vi "BonOMM-SAOMM.Test.vi"() -> ()   [LabVIEW 2011] (continued)
                n3227 = Array To Spreadsheet String(delimiter (Tab)="\n", array=w7372, 3:"%5f") -> (spreadsheet string=w7370:string)
                n3228 = Get Date/Time String(date format (0)=enum16{"short", "long", "abbreviated"}."short", want seconds? (F)=TRUE) -> (date string=w7356:string, time string=w7351:string)  [unwired: 1 in]
                n3229 = local read "path_syslogs"() -> (w7366:path)
                n3230 = Search and Replace String(replace all?=TRUE ("replace all? (F)"), input string=w7356, search string="-") -> (result string=w7350:string)  [unwired: 5 in, 3 out]
                n3231 = Search and Replace String(replace all?=TRUE ("replace all? (F)"), input string=w7351, search string=":") -> (result string=w7349:string)  [unwired: 5 in, 3 out]
                n3232 = Concatenate Strings(w7368, "\n\n***\n\n", w7370) -> (w7367:string)
                n3233 = Concatenate Strings(w7350, w7349, ".lvdt" ("name or relative path")) -> (w7359:string)
                n3234 = Build Path(base path=w7366, name or relative path="LVDTs") -> (appended path=w7364:path)
                n3235 = local read "File I/O Error"() -> (w7358:errorcluster)
                n3236 = Build Path(base path=w7364, name or relative path=w7359) -> (appended path=w7363:path)
                n3237 = Write to Text File(file (use dialog)=w7363, text=w7367, error in=w7358) -> (error out=w7357:errorcluster)  [unwired: 1 in, 2 out]
                n3238 = local write "File I/O Error"(w7357) -> ()
              }
              event "SpliterSelector": Value Change {
                n3239 = event-data() -> ("OldVal"=w7375:u16, "NewVal"=w7374:u16)  [unwired: 1 in, 3 out]
                n3240 = Not Equal?(x=w7375, y=w7374) -> (x != y?=w7373:bool)
                n3241 = case shown="True" w7373 {
                  frame False {
                  }
                  frame True {
                    n3242 = flat-sequence {
                      frame #0 {
                        "SplitterMoving" <- TRUE
                      }
                      frame #1 {
                        n3243 = flat-sequence {
                          tunnel: "SpliterSelector" -> [w7382]
                          frame #0 {
                            n3244 = case shown="1" w7382 {
                              tunnel: [w7383 w7388 w7389] -> _
                              frame 2 {
                                w7385 = u16 1 items=["Initialisation", "Mise dans le faisceau", "Retirer du faisceau"] ("Commande")
                                n3245 = local read "Splitter VRN"() -> (w7384:refnum<visa-resource-name>)
                                n3246 = call "MicroSlide-Execute.vi"("VISA resource name"=w7384, "Commande"=w7385) -> ("Error OUT"=w7383:errorcluster)  [unwired: 10 in, 3 out]
                              }
                              frame 0, Default {
                                w7386 = u16 0 items=["Initialisation", "Mise dans le faisceau", "Retirer du faisceau"] ("Commande")
                                n3247 = local read "Splitter VRN"() -> (w7387:refnum<visa-resource-name>)
                                n3248 = call "MicroSlide-Execute.vi"("VISA resource name"=w7387, "Commande"=w7386) -> ("Error OUT"=w7388:errorcluster)  [unwired: 10 in, 3 out]
                              }
                              frame 1 {
                                w7391 = u16 2 items=["Initialisation", "Mise dans le faisceau", "Retirer du faisceau"] ("Commande")
                                n3249 = local read "Splitter VRN"() -> (w7390:refnum<visa-resource-name>)
                                n3250 = call "MicroSlide-Execute.vi"("VISA resource name"=w7390, "Commande"=w7391) -> ("Error OUT"=w7389:errorcluster)  [unwired: 10 in, 3 out]
                              }
                            }
                          }
                          frame #1 {
                            n3251 = local write "SplitterMoving"(FALSE ("SplitterMoving")) -> ()
                          }
                        }
                        n3252 = while {
                          stop <- w7381 continue-if-true
                          n3253 = local read "SpliterIndic"() -> (w7378:bool)
                          n3254 = Wait (ms)(milliseconds to wait=u32 250) -> ()  [unwired: 1 out]
                          n3255 = Not(x=w7378) -> (.not. x?=→"SpliterIndic":bool)
                          n3256 = local read "SplitterMoving"() -> (w7381:bool)
                        }
                      }
                      frame #2 {
                        # "À mettre en gestion d'erreur"
                        n3257 = local write "SpliterIndic"(TRUE ("SpliterIndic")) -> ()
                      }
                    }
                  }
                }
              }
            }
          }
          "Événements Usagés" <- w956
          n3258 = while {
            stop <- w991 stop-if-true
            # "Boucle d'analyse d'image à haute fréquence ..."
            n3259 = event shown="[1] \"ProcessImage\": Value Change" {
              selector: _ -> [_ _]
              dyn-events: _ -> [_ _]
              timeout: 50 -> [_ _]
              event Timeout {
                n3260 = event-data() -> ()  [unwired: 1 in, 2 out]
              }
              event "ProcessImage": Value Change {
                n3261 = event-data() -> ()  [unwired: 1 in, 5 out]
                n3262 = local read "ROIXOffset"() -> (w999:u16)
                n3263 = local read "ROIYOffset"() -> (w995:u16)
                n3264 = local write "ProcessImage"(FALSE) -> ()
                n3265 = local read "XCentroid"() -> (w1000:dbl)
                n3266 = local read "YCentroid"() -> (w996:dbl)
                n3267 = local read "ImageBuffer"() -> (w1012:u16[][])
                n3268 = local read "MaskObjet"() -> (w1013:u8[][])
                n3269 = To Double Precision Float(number=w999) -> (double precision float=w998:dbl)
                n3270 = To Double Precision Float(number=w995) -> (double precision float=w997:dbl)
                n3271 = Subtract(x=w1000, y=w998) -> (x-y=w993:dbl)
                n3272 = Subtract(x=w996, y=w997) -> (x-y=w994:dbl)
                n3273 = local read "PixScale1"() -> (w1015:dbl)
                n3274 = local read "Binning"() -> (w1016:u16)
                n3275 = call "SAOMM-ROI-Stats.vi"("ImageBuffer"=w1012, "ObjectMask"=w1013, "intervals"=32) -> ("ROI Histogram"=→"Histogramme de la ROI":T10, "ImageStat"=w1009:T2)  [unwired: 11 in]
                "ImageStat" <- w1009
                n3276 = To Long Integer(number=w1012) -> (32bit integer=w1002:i32[][])
                n3277 = To Double Precision Float(number=w1016) -> (double precision float=w1014:dbl)
                n3278 = Multiply(x=w1015, y=w1014) -> (x*y=w1004:dbl)
                n3279 = call "PSF-Fitting.vi"("Centoid X"=w993, "Centroid Y"=w994, "ROI"=w1002, "''/pix"=w1004) -> ("Credible?"=w992:bool, "PSF Graph"=w1001:cluster{"PSF X":dbl[], "PSF Y":dbl[]}[], "Seeing"=w1003:dbl)  [unwired: 8 in, 1 out]
                n3280 = case shown="False" w992 {
                  tunnel: w1001 -> [_ w1025]
                  tunnel: w1003 -> [_ w1024]
                  tunnel: [w1019 w1025] -> w1011
                  tunnel: [inf w1024] -> w1010
                  frame False {
                    n3281 = Build Array(0.0) -> (w1021:dbl[])
                    n3282 = Bundle(w1021, w1021) -> (w1020:cluster{dbl[], dbl[]})  [unwired: 1 in]
                    n3283 = Build Array(w1020, w1020) -> (w1019:cluster{dbl[], dbl[]}[])
                  }
                  frame True {
                  }
                }
                "PSF Graph" <- w1011
                "Seeing" <- w1010
                n3284 = Unbundle By Name(w1009) -> ("ObjectMaximumValue"=w1008:dbl)
                n3285 = Greater?(x=w1008, y=50000.0) -> (0:w1006:bool)
                n3286 = property on="Saturé" class="Bool (strict)"("Blinking"=w1006, "Visible"=w1006) -> ()  [unwired: 2 in, 2 out]
              }
            }
            n3287 = local read "Quit"() -> (w991:bool)
          }
          n3288 = control-ref of="PrAMS actif"() -> (w958:refnum<vi>)
          n3289 = Tick Count (ms)() -> (millisecond timer value=w959:u32)
          n3290 = Tick Count (ms)() -> (millisecond timer value=w960:u32)
          n3291 = control-ref of="HexaCons actif"() -> (w957:refnum<vi>)
          n3292 = while {
            tunnel: [w1369] -> w949
            i -> [w1370]
            stop <- w1369 stop-if-true
            n3293 = event shown="[0] Timeout" {
              selector: _ -> [_ _ _ _ _ _ _ _ _ _ _ _ _ _ _ _ _ _ _ _ _ _ _]
              dyn-events: _ -> [_ _ _ _ _ _ _ _ _ _ _ _ _ _ _ _ _ _ _ _ _ _ _]
              timeout: 200 -> [_ _ _ _ _ _ _ _ _ _ _ _ _ _ _ _ _ _ _ _ _ _ _]
              tunnel: w1370 -> [w1378 _ _ _ _ _ _ _ _ _ _ _ _ _ _ _ _ _ _ _ _ _ _]
              event Timeout {
                # "À passer dans une boucle à part ?"
                n3294 = event-data() -> ()  [unwired: 1 in, 2 out]
                n3295 = local read "Integrating"() -> (w1375:bool)
                n3296 = Quotient & Remainder(x=w1378, y=25) -> (x-y*floor(x/y)=w1376:i32)  [unwired: 1 out]
                n3297 = Equal To 0?(x=w1378) -> (x = 0?=w1380:bool)
                n3298 = Equal To 0?(x=w1376) -> (x = 0?=w1374:bool)
                n3299 = Not(x=w1375) -> (.not. x?=w1373:bool)
                n3300 = And(x=w1374, y=w1373) -> (x .and. y?=w1372:bool)
                n3301 = Or(x="FalconRefresh", y=w1380) -> (x .or. y?=w1385:bool)
                n3302 = Equal?(x=w1378, y=1) -> (x = y?=w1382:bool)
                n3303 = Compound Arithmetic op=OR(w1382, "HexapodRefresh", w1372) -> (w1379:bool)
                n3304 = case shown="False" w1385 {
                  frame False {
                  }
                  frame True {
                    n3305 = Tick Count (ms)() -> (millisecond timer value=→"FalconQuery":u32)
                    n3306 = local write "FalconRefresh"(FALSE ("Refresh")) -> ()
                    n3307 = local read "PrAMS VRN"() -> (w1402:refnum<visa-resource-name>)
                    n3308 = local read "PrAMS Error"() -> (w1404:errorcluster)
                    n3309 = local read "MessageType"() -> (w1399:cluster{string[], u32[]})
                    n3310 = control-ref of="PrAMS actif"() -> (w1400:refnum<vi>)
                    n3311 = local read "Signature"() -> (w1398:u32)
                    n3312 = call "SAOMM-QueryFalcon.vi"("PRAMMS-COMM IN"=w1402, "Bool Refnum"=w1400, "Signature"=w1398, "Error IN"=w1404, "CommandCluster"=w1399) -> ("PRAMMS-COMM OUT"=w1401:refnum<visa-resource-name>, "Error OUT"=w1403:errorcluster)  [unwired: 9 in]
                    n3313 = local write "PrAMS Error"(w1403) -> ()
                    n3314 = local write "PrAMS VRN"(w1401) -> ()
                    "QueryingPraMS" <- TRUE
                  }
                }
                n3315 = case shown="False" w1379 {
                  frame False {
                  }
                  frame True {
                    n3316 = local write "HexapodRefresh"(FALSE ("Refresh")) -> ()
                    n3317 = Tick Count (ms)() -> (millisecond timer value=→"HexapodQuery":u32)
                    n3318 = local read "MessageType"() -> (w1391:cluster{string[], u32[]})
                    n3319 = control-ref of="HexaCons actif"() -> (w1387:refnum<vi>)
                    n3320 = local read "PrAMS Error"() -> (w1393:errorcluster)
                    n3321 = local read "Signature"() -> (w1390:u32)
                    n3322 = call "SAOMM-QueryHexapod.vi"("PRAMMS-COMM IN"="Hexapod VRN", "Bool Refnum"=w1387, "Signature"=w1390, "Error IN"=w1393, "EnumMessageType"=w1391) -> ("PRAMMS-COMM OUT"=w1388:refnum<visa-resource-name>, "Error OUT"=w1392:errorcluster)  [unwired: 9 in]
                    n3323 = local write "PrAMS Error"(w1392) -> ()
                    n3324 = local write "Hexapod VRN"(w1388) -> ()
                    "QueryingHexapod" <- TRUE ("Refresh")
                  }
                }
              }
              event "refresh": Value Change {
                n3325 = event-data() -> ()  [unwired: 1 in, 5 out]
                n3326 = case shown="True" "refresh" {
                  frame False {
                  }
                  frame True {
                    n3327 = flat-sequence {
                      frame #0 {
                        n3328 = local read "MessageType"() -> (w1414:cluster{string[], u32[]})
                        n3329 = control-ref of="PrAMS actif"() -> (w1413:refnum<vi>)
                        n3330 = local read "PrAMS VRN"() -> (w1412:refnum<visa-resource-name>)
                        n3331 = local read "PrAMS Error"() -> (w1411:errorcluster)
                        n3332 = local read "Signature"() -> (w1410:u32)
                        n3333 = call "SAOMM-SendGET.vi"("PRAMMS-COMM IN"=w1412, "Bool Refnum"=w1413, "MessageType"=w1414, "Signature"=w1410, "Error IN"=w1411, "Active GET"="GetCommand") -> ("PRAMMS-COMM OUT"=w1409:refnum<visa-resource-name>, "Error OUT"=w1408:errorcluster)  [unwired: 8 in]
                        n3334 = local write "PrAMS Error"(w1408) -> ()
                        n3335 = local write "PrAMS VRN"(w1409) -> ()
                      }
                      frame #1 {
                        n3336 = local write "refresh"(FALSE) -> ()
                      }
                    }
                  }
                }
              }
              event "Mode": Value Change {
                # "C'est ici qu'on changera les mutex pour les boutons quand ceux-ci seront définis ..."
                n3337 = event-data() -> ("OldVal"=w1417:u16, "NewVal"=w1416:u16)  [unwired: 1 in, 3 out]
                n3338 = case shown="2" w1417 {
                  frame 0, Default {
                    # "On passe de 'Opération fixe' à ..."
                  }
                  frame 1 {
                    # "On passe de 'Asservissement passif' à ..."
                  }
                  frame 2 {
                    # "On passe de 'Asservissement actif' à ..."
                  }
                  frame 3 {
                    # "On passe de 'Calibration' à ..."
                  }
                }
                n3339 = case shown="3" w1416 {
                  frame 0, Default {
                    # "... 'Opération fixe'"
                  }
                  frame 1 {
                    # "'Asservissement passif'"
                  }
                  frame 2 {
                    # "'Asservissement actif'"
                  }
                  frame 3 {
                    # "'Calibration'"
                  }
                }
              }
              event "ImgArray": Mouse Down {
                n3340 = event-data() -> ("Coords"=w1422:T48)  [unwired: 1 in, 6 out]
                n3341 = local read "Integrating"() -> (w1420:bool)
                n3342 = local read "Servo"() -> (w1419:bool)
                n3343 = Not(x=w1419) -> (.not. x?=w1418:bool)
                n3344 = And(x=w1420, y=w1418) -> (x .and. y?=w1421:bool)
                n3345 = case shown="True" w1421 {
                  tunnel: w1422 -> [_ w1457]
                  tunnel: w1418 -> [w1423 _]
                  frame False {
                    n3346 = case shown="False" w1423 {
                      frame False {
                        n3347 = One Button Dialog(message="Vous ne pouvez pas modifier la ROI pendant l'asservissement") -> ()  [unwired: 1 in, 1 out]
                      }
                      frame True {
                      }
                    }
                  }
                  frame True {
                    n3348 = control-ref of="ImgArray"() -> (w1454:refnum<vi>)
                    n3349 = local read "ROIWidth"() -> (w1453:u16)
                    n3350 = local read "ROIHeight"() -> (w1452:u16)
                    n3351 = call "Click2CursorPosition.vi"("reference"=w1454, "ClickPosition"=w1457) -> ("CursorX"=w1456:dbl, "CursorY"=w1455:dbl)  [unwired: 12 in]
                    n3352 = call "SAOMM-Cursor2ROI.vi"("ImgRef"=w1454, "CursorX"=w1456, "CursorY"=w1455, "ROIWidth"=w1453, "ROIHeight"=w1452) -> ("XÉtoile"=w1430:dbl, "YÉtoile"=w1429:dbl, "ROIXOffset"=w1434:u16, "ROIYOffset"=w1433:u16)  [unwired: 7 in]
                    n3353 = local write "YROIRef"(w1430) -> ()
                    n3354 = local write "XROIRef"(w1429) -> ()
                    n3355 = local write "ROIXOffset"(w1434) -> ()
                    n3356 = local write "ROIYOffset"(w1433) -> ()
                    n3357 = local read "Binning"() -> (w1443:u16)
                    n3358 = local read "ROIWidth"() -> (w1436:u16)
                    n3359 = local read "ROIHeight"() -> (w1437:u16)
                    n3360 = local read "Naxis1"() -> (w1441:u16)
                    n3361 = local read "Naxis2"() -> (w1440:u16)
                    n3362 = Bundle("XÉtoile"=w1430, "YÉtoile"=w1429) -> (w1435:cluster{"XÉtoile":dbl, "YÉtoile":dbl})  [unwired: 1 in]
                    n3363 = Bundle("Naxis1"=w1441, "Naxis2"=w1440) -> (w1442:cluster{"Naxis1":u16, "Naxis2":u16})  [unwired: 1 in]
                    n3364 = Bundle("ROIWidth"=w1436, "ROIHeight"=w1437) -> (w1439:cluster{"ROIWidth":u16, "ROIHeight":u16})  [unwired: 1 in]
                    n3365 = Bundle("ROIXOffset"=w1434, "ROIYOffset"=w1433) -> (w1438:cluster{"ROIXOffset":u16, "ROIYOffset":u16})  [unwired: 1 in]
                    n3366 = local read "MessageType"() -> (w1445:cluster{string[], u32[]})
                    n3367 = control-ref of="PrAMS-ACK"() -> (w1446:refnum<vi>)
                    n3368 = control-ref of="PrAMS actif"() -> (w1451:refnum<vi>)
                    n3369 = local read "PrAMS VRN"() -> (w1450:refnum<visa-resource-name>)
                    n3370 = local read "PrAMS Error"() -> (w1449:errorcluster)
                    n3371 = call "SAOMM-ROI_Fixer.vi"("Binning"=w1443, "Use Offset?"=TRUE, "naxis"=w1442, "ROI"=w1439, "Offset"=w1438, "Reference Pixel"=w1435) -> ("FixedOffset"=w1427:cluster{"ROIXOffset":u16, "ROIYOffset":u16}, "FixedPixel"=w1428:cluster{"PixelX":dbl, "PixelY":dbl})  [unwired: 6 in, 2 out]
                    n3372 = Unbundle By Name(w1428) -> ("PixelX"=w1426:dbl, "PixelY"=w1425:dbl)
                    n3373 = call "SAOMM-UpdateROI.vi"("PRAMMS-COMM IN"=w1450, "Active Refnum"=w1451, "PrAMS-ACK"=w1446, "MessageType"=w1445, "Error IN"=w1449, "Position"=w1427) -> ("PRAMMS-COMM OUT"=w1448:refnum<visa-resource-name>, "Error OUT"=w1447:errorcluster)  [unwired: 7 in, 1 out]
                    n3374 = local write "PrAMS Error"(w1447) -> ()
                    n3375 = local write "PrAMS VRN"(w1448) -> ()
                    n3376 = property on="ImgArray" class="IntGraph (strict)"() -> ("Cursor.Cursor Position"=w1432:T44)  [unwired: 2 in, 2 out]
                    n3377 = local write "XReference"(w1426) -> ()
                    n3378 = local write "YReference"(w1425) -> ()
                    n3379 = Bundle(cluster=w1432, "Cursor X"=w1426, "Cursor Y"=w1425) -> (w1431:T44)
                    n3380 = property on="ImgArray" class="IntGraph (strict)"("Cursor.Cursor Position"=w1431) -> ()  [unwired: 2 in, 2 out]
                  }
                }
              }
              event "ClearDump": Value Change {
                # "Tout ceci est du débuggage ..."
                n3381 = event-data() -> ()  [unwired: 1 in, 5 out]
                n3382 = local write "nDumped"(0 ("nDumped")) -> ()
                n3383 = local write "Dump"("") -> ()
              }
              event "ImageFPS": Value Change {
                n3384 = event-data() -> ()  [unwired: 1 in, 5 out]
                n3385 = flat-sequence {
                  tunnel: [w1462] -> w1461
                  tunnel: [w1465] -> w1460
                  tunnel: w1461 -> [w1465]
                  tunnel: w1460 -> [w1477]
                  frame #0 {
                    n3386 = Tick Count (ms)() -> (millisecond timer value=w1462:u32)
                  }
                  frame #1 {
                    n3387 = local read "MessageType"() -> (w1468:cluster{string[], u32[]})
                    n3388 = control-ref of="PrAMS actif"() -> (w1470:refnum<vi>)
                    n3389 = control-ref of="PrAMS-ACK"() -> (w1469:refnum<vi>)
                    n3390 = local read "PrAMS Error"() -> (w1471:errorcluster)
                    n3391 = local read "PrAMS VRN"() -> (w1472:refnum<visa-resource-name>)
                    n3392 = local read "ImageFPS"() -> (w1463:dbl)
                    n3393 = local read "Signature"() -> (w1464:u32)
                    n3394 = call-poly "SAOMM-Num2littleEndian.vi"("Number"=w1463) -> ("LiitleEndianedData"=w1466:u8[])  [unwired: 14 in]
                    n3395 = call "SAOMM-SendSET.vi"("PRAMMS-COMM IN"=w1472, "Active Refnum"=w1470, "PrAMS-ACK"=w1469, "Signature"=w1464, "Error IN"=w1471, "MessageType"=w1468, "Active SET"="emtSetImageDisplayFrameRate", "Value (little endianed byte array)"=w1466) -> ("PRAMMS-COMM OUT"=w1474:refnum<visa-resource-name>, "Error OUT"=w1473:errorcluster)  [unwired: 4 in, 2 out]
                    n3396 = local write "PrAMS Error"(w1473) -> ()
                    n3397 = local write "PrAMS VRN"(w1474) -> ()
                  }
                  frame #2 {
                    n3398 = Tick Count (ms)() -> (millisecond timer value=w1476:u32)
                    n3399 = Subtract(x=w1476, y=w1477) -> (x-y=→"SetFPSTime":u32)
                  }
                }
              }
              event "exptime": Value Change {
                n3400 = event-data() -> ()  [unwired: 1 in, 5 out]
                n3401 = flat-sequence {
                  tunnel: [w1480] -> w1479
                  tunnel: [w1482] -> w1478
                  tunnel: w1479 -> [w1482]
                  tunnel: w1478 -> [w1497]
                  frame #0 {
                    n3402 = Tick Count (ms)() -> (millisecond timer value=w1480:u32)
                  }
                  frame #1 {
                    n3403 = local read "MessageType"() -> (w1488:cluster{string[], u32[]})
                    n3404 = control-ref of="PrAMS actif"() -> (w1490:refnum<vi>)
                    n3405 = control-ref of="PrAMS-ACK"() -> (w1489:refnum<vi>)
                    n3406 = local read "PrAMS Error"() -> (w1491:errorcluster)
                    n3407 = local read "PrAMS VRN"() -> (w1492:refnum<visa-resource-name>)
                    n3408 = expression code="x*1000"("exptime") -> (w1484:dbl)
                    n3409 = local read "Signature"() -> (w1481:u32)
                    n3410 = To Unsigned Long Integer(number=w1484) -> (unsigned 32bit integer=w1483:u32)
                    n3411 = call-poly "SAOMM-Num2littleEndian.vi"("Number"=w1483) -> ("LiitleEndianedData"=w1486:u8[])  [unwired: 14 in]
                    n3412 = call "SAOMM-SendSET.vi"("PRAMMS-COMM IN"=w1492, "Active Refnum"=w1490, "PrAMS-ACK"=w1489, "Signature"=w1481, "Error IN"=w1491, "MessageType"=w1488, "Active SET"="emtSetImageExposureTime", "Value (little endianed byte array)"=w1486) -> ("PRAMMS-COMM OUT"=w1494:refnum<visa-resource-name>, "Error OUT"=w1493:errorcluster)  [unwired: 4 in, 2 out]
                    n3413 = local write "PrAMS Error"(w1493) -> ()
                    n3414 = local write "PrAMS VRN"(w1494) -> ()
                  }
                  frame #2 {
                    n3415 = Tick Count (ms)() -> (millisecond timer value=w1496:u32)
                    n3416 = Subtract(x=w1496, y=w1497) -> (x-y=→"SetExpTime":u32)
                  }
                }
              }
              event "FPGA Value": Value Change {
                n3417 = event-data() -> ("NewVal"=w1501:u16)  [unwired: 1 in, 4 out]
                n3418 = local read "Integrating"() -> (w1498:bool)
                n3419 = local read "Servo"() -> (w1499:bool)
                n3420 = Or(x=w1499, y=w1498) -> (x .or. y?=w1500:bool)
                n3421 = case shown="False" w1500 {
                  tunnel: w1501 -> [w1506 _]
                  frame False {
                    n3422 = Number To Decimal String(number=w1506) -> (decimal integer string=w1505:string)  [unwired: 1 in]
                    n3423 = call-poly "SAOMM-Num2littleEndian.vi"("Number"=w1506) -> ("LiitleEndianedData"=w1509:u8[])  [unwired: 14 in]
                    n3424 = local read "MessageType"() -> (w1512:cluster{string[], u32[]})
                    n3425 = control-ref of="PrAMS actif"() -> (w1514:refnum<vi>)
                    n3426 = control-ref of="PrAMS-ACK"() -> (w1513:refnum<vi>)
                    n3427 = local read "PrAMS VRN"() -> (w1516:refnum<visa-resource-name>)
                    n3428 = local read "PrAMS Error"() -> (w1515:errorcluster)
                    n3429 = control-ref of="TERMINAL"() -> (w1507:refnum<vi>)
                    n3430 = control-ref of="Indicateur d'état"() -> (w1508:refnum<vi>)
                    n3431 = local read "Signature"() -> (w1510:u32)
                    n3432 = Concatenate Strings("FAPG.set -> (", w1505, ")") -> (w1503:string)
                    n3433 = call "TERMINAL.vi"("Indicateur Refnum"=w1508, "Terminal Refnum"=w1507, "Indicateur d'état"=w1503) -> ()
                    n3434 = call "SAOMM-SendSET.vi"("PRAMMS-COMM IN"=w1516, "Active Refnum"=w1514, "PrAMS-ACK"=w1513, "Signature"=w1510, "Error IN"=w1515, "MessageType"=w1512, "Active SET"="emtSetFPGACtrl", "Value (little endianed byte array)"=w1509) -> ("PRAMMS-COMM OUT"=w1518:refnum<visa-resource-name>, "Error OUT"=w1517:errorcluster)  [unwired: 4 in, 2 out]
                    n3435 = local write "PrAMS Error"(w1517) -> ()
                    n3436 = local write "PrAMS VRN"(w1518) -> ()
                  }
                  frame True {
                    n3437 = One Button Dialog(message="Impossible de modifier le FPGActrl pendant que la caméra fonctionne") -> ()  [unwired: 1 in, 1 out]
                  }
                }
              }
              event "Binning": Value Change {
                n3438 = event-data() -> ("OldVal"=w1524:u16, "NewVal"=w1523:u16)  [unwired: 1 in, 3 out]
                n3439 = local read "Integrating"() -> (w1521:bool)
                n3440 = local read "Servo"() -> (w1520:bool)
                n3441 = Or(x=w1521, y=w1520) -> (x .or. y?=w1522:bool)
                n3442 = case shown="False" w1522 {
                  tunnel: w1524 -> [w1536 _]
                  tunnel: w1523 -> [w1534 _]
                  frame False {
                    w1548 = "cam_Binning "
                    # "Passer dans une astrométrie ?"
                    n3443 = flat-sequence {
                      tunnel: [w1581] -> w1564
                      tunnel: [w1597] -> w1563
                      tunnel: w1564 -> [w1597]
                      tunnel: w1535 -> [w1589]
                      tunnel: w1533 -> [w1588]
                      tunnel: w1532 -> [w1587]
                      tunnel: [w1586] -> w1562
                      tunnel: [w1585] -> w1561
                      tunnel: [w1584] -> w1560
                      tunnel: w1563 -> [w1611]
                      tunnel: [w1608] -> w1531
                      tunnel: w1562 -> [w1608]
                      tunnel: w1561 -> [w1607]
                      tunnel: w1560 -> [w1602]
                      frame #0 {
                        n3444 = Tick Count (ms)() -> (millisecond timer value=w1581:u32)
                      }
                      frame #1 {
                        n3445 = local read "MessageType"() -> (w1591:cluster{string[], u32[]})
                        n3446 = control-ref of="PrAMS-ACK"() -> (w1582:refnum<vi>)
                        n3447 = control-ref of="PrAMS actif"() -> (w1583:refnum<vi>)
                        n3448 = local read "Signature"() -> (w1590:u32)
                        n3449 = local read "PrAMS VRN"() -> (w1596:refnum<visa-resource-name>)
                        n3450 = local read "PrAMS Error"() -> (w1595:errorcluster)
                        n3451 = call "SAOMM-BinningFixer.vi"("PRAMMS-COMM IN"=w1596, "Active Refnum"=w1583, "PrAMS-ACK"=w1582, "Signature"=w1590, "SendSET"=TRUE, "MessageType"=w1591, "Error IN"=w1595, "Binning"=w1589, "NAXIS"=w1587, "ROI Sizes"=w1588) -> ("PRAMMS-COMM OUT"=w1594:refnum<visa-resource-name>, "ScaleFactor"=w1586:dbl, "ROISizesOut"=w1585:T49, "ROIMinMax"=w1584:T50, "Error OUT"=w1593:errorcluster)  [unwired: 1 in]
                        n3452 = local write "PrAMS Error"(w1593) -> ()
                        n3453 = local write "PrAMS VRN"(w1594) -> ()
                      }
                      frame #2 {
                        n3454 = Tick Count (ms)() -> (millisecond timer value=w1610:u32)
                        n3455 = Subtract(x=w1610, y=w1611) -> (x-y=→"SetBinningTime":u32)
                        n3456 = Unbundle(w1607) -> ("ROIXOffset OUT"=w1606:u16, "ROIYOffset OUT"=w1605:u16, "ROIWidth OUT"=w1604:u16, "ROIHeight OUT"=w1603:u16)
                        n3457 = Unbundle(w1602) -> ("ROIXMin"=→"ROIXMin":u16, "ROIYXMax"=→"ROIXMax":u16, "ROIYMin"=→"ROIYMin":u16, "ROIYMax"=→"ROIYMax":u16)
                        n3458 = local write "ROIXOffset"(w1606) -> ()
                        n3459 = local write "ROIYOffset"(w1605) -> ()
                        n3460 = local write "ROIWidth"(w1604) -> ()
                        n3461 = local write "ROIHeight"(w1603) -> ()
                      }
                    }
                    n3462 = local read "Naxis1"() -> (w1525:u16)
                    n3463 = local read "Naxis2"() -> (w1526:u16)
                    n3464 = local read "ROIXOffset"() -> (w1530:u16)
                    n3465 = local read "ROIYOffset"() -> (w1529:u16)
                    n3466 = local read "ROIWidth"() -> (w1528:u16)
                    n3467 = local read "ROIHeight"() -> (w1527:u16)
                    n3468 = Bundle("OldVal"=w1536, "NewVal"=w1534) -> (w1535:cluster{"OldVal":u16, "NewVal":u16})  [unwired: 1 in]
                    n3469 = Bundle("Naxis1"=w1525, "Naxis2"=w1526) -> (w1532:cluster{"Naxis1":u16, "Naxis2":u16})  [unwired: 1 in]
                    n3470 = Bundle("ROIXOffset"=w1530, "ROIYOffset"=w1529, "ROIWidth"=w1528, "ROIHeight"=w1527) -> (w1533:T51)  [unwired: 1 in]
                    n3471 = property on="ImgArray" class="IntGraph (strict)"() -> ("Cursor.Cursor X"=w1559:dbl, "Cursor.Cursor Y"=w1558:dbl)  [unwired: 2 in, 2 out]
                    n3472 = case shown="2" w1534 {
                      tunnel: [TRUE FALSE FALSE FALSE] -> w1540
                      tunnel: [FALSE TRUE FALSE FALSE] -> w1539
                      tunnel: [FALSE FALSE TRUE FALSE] -> w1538
                      tunnel: [FALSE FALSE FALSE TRUE] -> w1537
                      frame 1, Default {
                      }
                      frame 2 {
                      }
                      frame 4 {
                      }
                      frame 5 {
                      }
                    }
                    n3473 = Multiply(x=w1531, y=w1559) -> (x*y=w1557:dbl)
                    n3474 = Multiply(x=w1558, y=w1531) -> (x*y=w1556:dbl)
                    n3475 = Round To Nearest(number=w1557) -> (nearest integer value=w1555:dbl)
                    n3476 = Round To Nearest(number=w1556) -> (nearest integer value=w1554:dbl)
                    n3477 = Current VI's Menubar() -> (w1553:refnum<k9>)
                    n3478 = Concatenate Strings(w1548, "1x1" ("string")) -> (w1549:string)
                    n3479 = Set Menu Item Info(6:w1540, 7:w1549, 11:w1553) -> (3:w1552:refnum<k9>)  [unwired: 4 in, 1 out]
                    n3480 = Concatenate Strings(w1548, "2x2" ("string")) -> (w1543:string)
                    n3481 = Set Menu Item Info(6:w1539, 7:w1543, 11:w1552) -> (3:w1551:refnum<k9>)  [unwired: 4 in, 1 out]
                    n3482 = local write "YReference"(w1554) -> ()
                    n3483 = local write "XReference"(w1555) -> ()
                    n3484 = Concatenate Strings(w1548, "4x4" ("string")) -> (w1542:string)
                    n3485 = Set Menu Item Info(6:w1538, 7:w1542, 11:w1551) -> (3:w1550:refnum<k9>)  [unwired: 4 in, 1 out]
                    n3486 = Concatenate Strings(w1548, "5x5" ("string")) -> (w1541:string)
                    n3487 = property on="ImgArray" class="IntGraph (strict)"("Cursor.Cursor X"=w1555, "Cursor.Cursor Y"=w1554) -> ()  [unwired: 2 in, 2 out]
                    n3488 = Set Menu Item Info(6:w1537, 7:w1541, 11:w1550) -> ()  [unwired: 4 in, 2 out]
                  }
                  frame True {
                  }
                }
              }
              event "EMGain": Value Change {
                n3489 = event-data() -> ("NewVal"=w1615:u16)  [unwired: 1 in, 4 out]
                n3490 = local read "Integrating"() -> (w1613:bool)
                n3491 = local read "Servo"() -> (w1614:bool)
                n3492 = Or(x=w1614, y=w1613) -> (x .or. y?=w1612:bool)
                n3493 = case shown="False" w1612 {
                  tunnel: w1615 -> [w1616 _]
                  frame False {
                    n3494 = call-poly "SAOMM-Num2littleEndian.vi"("Number"=w1616) -> ("LiitleEndianedData"=w1617:u8[])  [unwired: 14 in]
                    n3495 = local read "MessageType"() -> (w1620:cluster{string[], u32[]})
                    n3496 = control-ref of="PrAMS actif"() -> (w1622:refnum<vi>)
                    n3497 = control-ref of="PrAMS-ACK"() -> (w1621:refnum<vi>)
                    n3498 = local read "PrAMS VRN"() -> (w1624:refnum<visa-resource-name>)
                    n3499 = local read "PrAMS Error"() -> (w1623:errorcluster)
                    n3500 = local read "Signature"() -> (w1618:u32)
                    n3501 = call "SAOMM-SendSET.vi"("PRAMMS-COMM IN"=w1624, "Active Refnum"=w1622, "PrAMS-ACK"=w1621, "Signature"=w1618, "Error IN"=w1623, "MessageType"=w1620, "Active SET"="emtSetImageEMGain", "Value (little endianed byte array)"=w1617) -> ("PRAMMS-COMM OUT"=w1626:refnum<visa-resource-name>, "Error OUT"=w1625:errorcluster)  [unwired: 4 in, 2 out]
                    n3502 = local write "PrAMS Error"(w1625) -> ()
                    n3503 = local write "PrAMS VRN"(w1626) -> ()
                  }
                  frame True {
                  }
                }
              }
              event "GoCam": Value Change {
                n3504 = event-data() -> ()  [unwired: 1 in, 5 out]
                n3505 = flat-sequence {
                  tunnel: [w1630] -> w1628
                  tunnel: [w1633] -> w1627
                  tunnel: w1628 -> [w1633]
                  tunnel: w1627 -> [w1644]
                  frame #0 {
                    n3506 = local write "GoCam"(FALSE ("GoCam")) -> ()
                    n3507 = Tick Count (ms)() -> (millisecond timer value=w1630:u32)
                  }
                  frame #1 {
                    # "emtStartAcquisition ne prend pas d'arguments"
                    n3508 = local read "MessageType"() -> (w1635:cluster{string[], u32[]})
                    n3509 = control-ref of="PrAMS actif"() -> (w1637:refnum<vi>)
                    n3510 = control-ref of="PrAMS-ACK"() -> (w1636:refnum<vi>)
                    n3511 = local read "PrAMS Error"() -> (w1638:errorcluster)
                    n3512 = local read "PrAMS VRN"() -> (w1639:refnum<visa-resource-name>)
                    n3513 = local read "Signature"() -> (w1631:u32)
                    n3514 = call "SAOMM-SendSET.vi"("PRAMMS-COMM IN"=w1639, "Active Refnum"=w1637, "PrAMS-ACK"=w1636, "Signature"=w1631, "Error IN"=w1638, "MessageType"=w1635, "Active SET"="emtStartAcquisition", "Value (little endianed byte array)"=u8[] []) -> ("PRAMMS-COMM OUT"=w1641:refnum<visa-resource-name>, "Error OUT"=w1640:errorcluster)  [unwired: 4 in, 2 out]
                    n3515 = local write "PrAMS Error"(w1640) -> ()
                    n3516 = local write "PrAMS VRN"(w1641) -> ()
                  }
                  frame #2 {
                    n3517 = Tick Count (ms)() -> (millisecond timer value=w1643:u32)
                    n3518 = Subtract(x=w1643, y=w1644) -> (x-y=→"StartTime":u32)
                  }
                }
              }
              event "StopCam": Value Change {
                n3519 = event-data() -> ()  [unwired: 1 in, 5 out]
                n3520 = flat-sequence {
                  tunnel: [w1648] -> w1646
                  tunnel: [w1651] -> w1645
                  tunnel: w1646 -> [w1651]
                  tunnel: w1645 -> [w1662]
                  frame #0 {
                    n3521 = local write "StopCam"(FALSE ("StopCam")) -> ()
                    n3522 = Tick Count (ms)() -> (millisecond timer value=w1648:u32)
                  }
                  frame #1 {
                    # "emtStartAcquisition ne prend pas d'arguments"
                    n3523 = local read "PrAMS VRN"() -> (w1657:refnum<visa-resource-name>)
                    n3524 = control-ref of="PrAMS-ACK"() -> (w1654:refnum<vi>)
                    n3525 = local read "PrAMS Error"() -> (w1656:errorcluster)
                    n3526 = local read "MessageType"() -> (w1653:cluster{string[], u32[]})
                    n3527 = control-ref of="PrAMS actif"() -> (w1655:refnum<vi>)
                    n3528 = local read "Signature"() -> (w1649:u32)
                    n3529 = call "SAOMM-SendSET.vi"("PRAMMS-COMM IN"=w1657, "Active Refnum"=w1655, "PrAMS-ACK"=w1654, "Signature"=w1649, "Error IN"=w1656, "MessageType"=w1653, "Active SET"="emtStopAcquisition", "Value (little endianed byte array)"=u8[] []) -> ("PRAMMS-COMM OUT"=w1659:refnum<visa-resource-name>, "Error OUT"=w1658:errorcluster)  [unwired: 4 in, 2 out]
                    n3530 = local write "PrAMS Error"(w1658) -> ()
                    n3531 = local write "PrAMS VRN"(w1659) -> ()
                  }
                  frame #2 {
                    n3532 = Tick Count (ms)() -> (millisecond timer value=w1661:u32)
                    n3533 = Subtract(x=w1661, y=w1662) -> (x-y=→"StopTime":u32)
                  }
                }
              }
              event "ROIsurface": Value Change {
                n3534 = event-data() -> ()  [unwired: 1 in, 5 out]
                n3535 = local read "Mode"() -> (w1665:u16)
                n3536 = local read "Servo"() -> (w1666:bool)
                n3537 = Equal?(x=w1665, y=u16 2) -> (x = y?=w1663:bool)
                n3538 = And(x=w1666, y=w1663) -> (x .and. y?=w1667:bool)
                n3539 = case shown="False" w1667 {
                  frame False {
                    w1679 = 0.0 ("y")
                    # "Pour l'instant, on met le pixel de référence au centre de la ROI"
                    # "Est-ce que le binning ne devrait pas apparaître ici ?!?"
                    n3540 = control-ref of="PrAMS-ACK"() -> (w1684:refnum<vi>)
                    n3541 = local read "MessageType"() -> (w1683:cluster{string[], u32[]})
                    n3542 = control-ref of="PrAMS actif"() -> (w1685:refnum<vi>)
                    n3543 = local read "Signature"() -> (w1689:u32)
                    n3544 = local read "PrAMS VRN"() -> (w1693:refnum<visa-resource-name>)
                    n3545 = local read "PrAMS Error"() -> (w1686:errorcluster)
                    n3546 = local read "ROISizes"() -> (w1699:u16[])
                    n3547 = call-poly "SAOMM-Num2littleEndian.vi"("Number"=w1679) -> ("LiitleEndianedData"=w1681:u8[])  [unwired: 14 in]
                    n3548 = call-poly "SAOMM-Num2littleEndian.vi"("Number"=w1679) -> ("LiitleEndianedData"=w1680:u8[])  [unwired: 14 in]
                    n3549 = Index Array(array=w1699, index="ROIsurface") -> (element=w1671:u16)
                    n3550 = call "SAOMM-SendSET.vi"("PRAMMS-COMM IN"=w1693, "Active Refnum"=w1685, "PrAMS-ACK"=w1684, "Signature"=w1689, "Error IN"=w1686, "MessageType"=w1683, "Active SET"="emtSetROIXReferencePoint", "Value (little endianed byte array)"=w1681) -> ("PRAMMS-COMM OUT"=w1695:refnum<visa-resource-name>, "Error OUT"=w1694:errorcluster)  [unwired: 4 in, 2 out]
                    n3551 = local write "ROIWidth"(w1671) -> ()
                    n3552 = local write "ROIHeight"(w1671) -> ()
                    n3553 = call-poly "SAOMM-Num2littleEndian.vi"("Number"=w1671) -> ("LiitleEndianedData"=w1703:u8[])  [unwired: 14 in]
                    n3554 = call "SAOMM-SendSET.vi"("PRAMMS-COMM IN"=w1695, "Active Refnum"=w1685, "PrAMS-ACK"=w1684, "Signature"=w1689, "Error IN"=w1694, "MessageType"=w1683, "Active SET"="emtSetROIYReferencePoint", "Value (little endianed byte array)"=w1680) -> ("PRAMMS-COMM OUT"=w1692:refnum<visa-resource-name>)  [unwired: 4 in, 3 out]
                    n3555 = call "SAOMM-SendSET.vi"("PRAMMS-COMM IN"=w1692, "Active Refnum"=w1685, "PrAMS-ACK"=w1684, "Signature"=w1689, "MessageType"=w1683, "Active SET"="emtSetROIWidth", "Value (little endianed byte array)"=w1703) -> ("PRAMMS-COMM OUT"=w1702:refnum<visa-resource-name>, "Error OUT"=w1701:errorcluster)  [unwired: 5 in, 2 out]
                    n3556 = call "SAOMM-SendSET.vi"("PRAMMS-COMM IN"=w1702, "Active Refnum"=w1685, "PrAMS-ACK"=w1684, "Signature"=w1689, "Error IN"=w1701, "MessageType"=w1683, "Active SET"="emtSetROIHeight", "Value (little endianed byte array)"=w1703) -> ("PRAMMS-COMM OUT"=w1691:refnum<visa-resource-name>, "Error OUT"=w1688:errorcluster)  [unwired: 4 in, 2 out]
                    n3557 = To Double Precision Float(number=w1671) -> (double precision float=w1672:dbl)
                    n3558 = To Double Precision Float(number=w1671) -> (double precision float=w1670:dbl)
                    n3559 = expression code="x/2.0"(w1672) -> (w1669:dbl)
                    n3560 = expression code="x/2.0"(w1670) -> (w1668:dbl)
                    n3561 = local write "XROIRef"(w1669) -> ()
                    n3562 = local write "YROIRef"(w1668) -> ()
                    n3563 = call-poly "SAOMM-Num2littleEndian.vi"("Number"=w1669) -> ("LiitleEndianedData"=w1674:u8[])  [unwired: 14 in]
                    n3564 = call-poly "SAOMM-Num2littleEndian.vi"("Number"=w1668) -> ("LiitleEndianedData"=w1673:u8[])  [unwired: 14 in]
                    n3565 = call "SAOMM-SendSET.vi"("PRAMMS-COMM IN"=w1691, "Active Refnum"=w1685, "PrAMS-ACK"=w1684, "Signature"=w1689, "Error IN"=w1688, "MessageType"=w1683, "Active SET"="emtSetROIXReferencePoint", "Value (little endianed byte array)"=w1674) -> ("PRAMMS-COMM OUT"=w1696:refnum<visa-resource-name>, "Error OUT"=w1697:errorcluster)  [unwired: 4 in, 2 out]
                    n3566 = call "SAOMM-SendSET.vi"("PRAMMS-COMM IN"=w1696, "Active Refnum"=w1685, "PrAMS-ACK"=w1684, "Signature"=w1689, "Error IN"=w1697, "MessageType"=w1683, "Active SET"="emtSetROIYReferencePoint", "Value (little endianed byte array)"=w1673) -> ("PRAMMS-COMM OUT"=w1690:refnum<visa-resource-name>, "Error OUT"=w1687:errorcluster)  [unwired: 4 in, 2 out]
                    n3567 = local write "PrAMS Error"(w1687) -> ()
                    n3568 = local write "PrAMS VRN"(w1690) -> ()
                  }
                  frame True {
                  }
                }
              }
              event "UpdateROI": Value Change {
                n3569 = event-data() -> ()  [unwired: 1 in, 5 out]
                n3570 = local read "Servo"() -> (w1704:bool)
                n3571 = case shown="False" w1704 {
                  frame False {
                    n3572 = flat-sequence {
                      tunnel: [w1708] -> w1706
                      tunnel: [w1743] -> w1705
                      tunnel: w1706 -> [w1743]
                      tunnel: w1705 -> [w1746]
                      frame #0 {
                        n3573 = local write "UpdateROI"(FALSE) -> ()
                        n3574 = Tick Count (ms)() -> (millisecond timer value=w1708:u32)
                      }
                      frame #1 {
                        n3575 = local read "Binning"() -> (w1734:u16)
                        n3576 = local read "ROIWidth"() -> (w1725:u16)
                        n3577 = local read "ROIHeight"() -> (w1726:u16)
                        n3578 = local read "Naxis1"() -> (w1732:u16)
                        n3579 = local read "Naxis2"() -> (w1731:u16)
                        n3580 = local read "ROIXOffset"() -> (w1727:u16)
                        n3581 = local read "ROIYOffset"() -> (w1728:u16)
                        n3582 = local read "XROIRef"() -> (w1723:dbl)
                        n3583 = local read "YROIRef"() -> (w1722:dbl)
                        n3584 = Bundle("XROIRef"=w1723, "YROIRef"=w1722) -> (w1724:cluster{"XROIRef":dbl, "YROIRef":dbl})  [unwired: 1 in]
                        n3585 = Bundle("Naxis1"=w1732, "Naxis2"=w1731) -> (w1733:cluster{"Naxis1":u16, "Naxis2":u16})  [unwired: 1 in]
                        n3586 = Bundle("ROIWidth"=w1725, "ROIHeight"=w1726) -> (w1730:cluster{"ROIWidth":u16, "ROIHeight":u16})  [unwired: 1 in]
                        n3587 = Bundle("ROIXOffset"=w1727, "ROIYOffset"=w1728) -> (w1729:cluster{"ROIXOffset":u16, "ROIYOffset":u16})  [unwired: 1 in]
                        n3588 = call "SAOMM-ROI_Fixer.vi"("Binning"=w1734, "Use Offset?"=TRUE, "naxis"=w1733, "ROI"=w1730, "Offset"=w1729, "Reference Pixel"=w1724) -> ("FixedOffset"=w1711:cluster{"ROIXOffset":u16, "ROIYOffset":u16}, "FixedPixel"=w1709:cluster{"PixelX":dbl, "PixelY":dbl})  [unwired: 6 in, 2 out]
                        n3589 = Unbundle By Name(w1711) -> ("ROIXOffset"=w1721:u16, "ROIYOffset"=w1720:u16)
                        n3590 = local read "MessageType"() -> (w1736:cluster{string[], u32[]})
                        n3591 = control-ref of="PrAMS-ACK"() -> (w1737:refnum<vi>)
                        n3592 = control-ref of="PrAMS actif"() -> (w1742:refnum<vi>)
                        n3593 = local read "PrAMS VRN"() -> (w1741:refnum<visa-resource-name>)
                        n3594 = local read "PrAMS Error"() -> (w1740:errorcluster)
                        n3595 = Unbundle By Name(w1709) -> ("PixelX"=w1712:dbl, "PixelY"=w1715:dbl)
                        n3596 = Bundle("ROIYOffset"=w1720, "ROIXOffset"=w1721) -> (w1710:cluster{"ROIYOffset":u16, "ROIXOffset":u16})  [unwired: 1 in]
                        n3597 = local write "XReference"(w1712) -> ()
                        n3598 = local write "YReference"(w1715) -> ()
                        n3599 = To Double Precision Float(number=w1721) -> (double precision float=w1714:dbl)
                        n3600 = To Double Precision Float(number=w1720) -> (double precision float=w1713:dbl)
                        n3601 = call "SAOMM-UpdateROI.vi"("PRAMMS-COMM IN"=w1741, "Active Refnum"=w1742, "PrAMS-ACK"=w1737, "MessageType"=w1736, "Error IN"=w1740, "Position"=w1710) -> ("PRAMMS-COMM OUT"=w1739:refnum<visa-resource-name>, "Error OUT"=w1738:errorcluster)  [unwired: 7 in, 1 out]
                        n3602 = property on="ImgArray" class="IntGraph (strict)"() -> ("Cursor.Cursor Position"=w1719:T44)  [unwired: 2 in, 2 out]
                        n3603 = local write "PrAMS Error"(w1738) -> ()
                        n3604 = local write "PrAMS VRN"(w1739) -> ()
                        n3605 = Add(x=w1713, y=w1712) -> (x+y=w1716:dbl)
                        n3606 = Add(x=w1714, y=w1715) -> (x+y=w1717:dbl)
                        n3607 = Bundle(cluster=w1719, "Cursor X"=w1716, "Cursor Y"=w1717) -> (w1718:T44)
                        n3608 = property on="ImgArray" class="IntGraph (strict)"("Cursor.Cursor Position"=w1718) -> ()  [unwired: 2 in, 2 out]
                      }
                      frame #2 {
                        n3609 = Tick Count (ms)() -> (millisecond timer value=w1745:u32)
                        n3610 = Subtract(x=w1745, y=w1746) -> (x-y=→"SetROITime":u32)
                      }
                    }
                  }
                  frame True {
                    n3611 = local read "FIFO d'erreur"() -> (w1748:T7)
                    n3612 = call "Error_Format.vi"("FIFO IN"=w1748, "Source"="PrAMS", "Comment"="Impossible de modifier les paramères de la ROI pendant l'asserviseement.") -> ("FIFO OUT"=w1749:T7)  [unwired: 14 in, 2 out]
                    n3613 = local write "FIFO d'erreur"(w1749) -> ()
                  }
                }
              }
              event "Milieu": Value Change {
                # "Calcul les paramètres du milieu"
                n3614 = event-data() -> ()  [unwired: 1 in, 5 out]
                n3615 = local read "Binning"() -> (w1758:u16)
                n3616 = local read "ROIWidth"() -> (w1762:u16)
                n3617 = local read "ROIHeight"() -> (w1761:u16)
                n3618 = local read "Naxis1"() -> (w1759:u16)
                n3619 = local read "Naxis2"() -> (w1760:u16)
                n3620 = formula code="Xoff=((nax1/bin)-ROIw)/2;\nYoff=((nax2/bin)-ROIh)/2;"("bin"=w1758, "nax1"=w1759, "nax2"=w1760, "ROIw"=w1762, "ROIh"=w1761) -> ("Xoff"=w1757:dbl, "Yoff"=w1755:dbl)
                n3621 = local read "XROIRef"() -> (w1764:dbl)
                n3622 = local read "YROIRef"() -> (w1763:dbl)
                n3623 = local write "Milieu"(FALSE ("Use Offset?")) -> ()
                n3624 = Bundle("XROIRef"=w1764, "YROIRef"=w1763) -> (w1776:cluster{"XROIRef":dbl, "YROIRef":dbl})  [unwired: 1 in]
                n3625 = To Unsigned Word Integer(number=w1757) -> (unsigned 16bit integer=w1756:u16)
                n3626 = To Unsigned Word Integer(number=w1755) -> (unsigned 16bit integer=w1754:u16)
                n3627 = Bundle("Naxis1"=w1759, "Naxis2"=w1760) -> (w1779:cluster{"Naxis1":u16, "Naxis2":u16})  [unwired: 1 in]
                n3628 = Bundle("ROIWidth"=w1762, "ROIHeight"=w1761) -> (w1778:cluster{"ROIWidth":u16, "ROIHeight":u16})  [unwired: 1 in]
                n3629 = local write "ROIXOffset"(w1756) -> ()
                n3630 = local write "ROIYOffset"(w1754) -> ()
                n3631 = Bundle(w1756, w1754) -> (w1777:cluster{u16, u16})  [unwired: 1 in]
                n3632 = call "SAOMM-ROI_Fixer.vi"("Binning"=w1758, "Use Offset?"=TRUE, "naxis"=w1779, "ROI"=w1778, "Offset"=w1777, "Reference Pixel"=w1776) -> ("FixedOffset"=w1767:cluster{"ROIXOffset":u16, "ROIYOffset":u16}, "FixedPixel"=w1765:cluster{"PixelX":dbl, "PixelY":dbl})  [unwired: 6 in, 2 out]
                n3633 = local read "MessageType"() -> (w1781:cluster{string[], u32[]})
                n3634 = control-ref of="PrAMS-ACK"() -> (w1782:refnum<vi>)
                n3635 = control-ref of="PrAMS actif"() -> (w1787:refnum<vi>)
                n3636 = local read "PrAMS VRN"() -> (w1786:refnum<visa-resource-name>)
                n3637 = local read "PrAMS Error"() -> (w1785:errorcluster)
                n3638 = Unbundle By Name(w1767) -> ("ROIXOffset"=w1775:u16, "ROIYOffset"=w1774:u16)
                n3639 = Unbundle By Name(w1765) -> ("PixelX"=w1768:dbl, "PixelY"=w1771:dbl)
                n3640 = To Double Precision Float(number=w1775) -> (double precision float=w1770:dbl)
                n3641 = To Double Precision Float(number=w1774) -> (double precision float=w1769:dbl)
                n3642 = Bundle("ROIYOffset"=w1774, "ROIXOffset"=w1775) -> (w1766:cluster{"ROIYOffset":u16, "ROIXOffset":u16})  [unwired: 1 in]
                n3643 = property on="ImgArray" class="IntGraph (strict)"() -> ("Cursor.Cursor Position"=w1773:T44)  [unwired: 2 in, 2 out]
                n3644 = Add(x=w1769, y=w1768) -> (x+y=w1753:dbl)
                n3645 = Add(x=w1770, y=w1771) -> (x+y=w1752:dbl)
                n3646 = call "SAOMM-UpdateROI.vi"("PRAMMS-COMM IN"=w1786, "Active Refnum"=w1787, "PrAMS-ACK"=w1782, "MessageType"=w1781, "Error IN"=w1785, "Position"=w1766) -> ("PRAMMS-COMM OUT"=w1784:refnum<visa-resource-name>, "Error OUT"=w1783:errorcluster)  [unwired: 7 in, 1 out]
                n3647 = local write "PrAMS Error"(w1783) -> ()
                n3648 = local write "XReference"(w1753) -> ()
                n3649 = local write "PrAMS VRN"(w1784) -> ()
                n3650 = local write "YReference"(w1752) -> ()
                n3651 = Bundle(cluster=w1773, "Cursor X"=w1753, "Cursor Y"=w1752) -> (w1772:T44)
                n3652 = property on="ImgArray" class="IntGraph (strict)"("Cursor.Cursor Position"=w1772) -> ()  [unwired: 2 in, 2 out]
              }
              event "FalconProcessed": Value Change {
                n3653 = event-data() -> ()  [unwired: 1 in, 5 out]
                n3654 = case shown="True" "FalconProcessed" {
                  frame False {
                  }
                  frame True {
                    n3655 = local write "FalconProcessed"(FALSE ("FalconProcessed")) -> ()
                    n3656 = local read "Nb_FalconProc_demandé"() -> (w1789:u32)
                    n3657 = local read "MessageType"() -> (w1795:cluster{string[], u32[]})
                    n3658 = control-ref of="PrAMS actif"() -> (w1796:refnum<vi>)
                    n3659 = local read "PrAMS VRN"() -> (w1792:refnum<visa-resource-name>)
                    n3660 = local read "PrAMS Error"() -> (w1797:errorcluster)
                    n3661 = Increment(x=w1789) -> (x+1=→"Nb_FalconProc_demandé":u32)
                    n3662 = local read "Signature"() -> (w1793:u32)
                    n3663 = call "SAOMM-SendGET.vi"("PRAMMS-COMM IN"=w1792, "Bool Refnum"=w1796, "MessageType"=w1795, "Signature"=w1793, "Error IN"=w1797, "Active GET"="emtGetProcessedFalconImage" ("Active SET")) -> ("PRAMMS-COMM OUT"=w1791:refnum<visa-resource-name>, "Error OUT"=w1798:errorcluster)  [unwired: 8 in]
                    n3664 = local write "PrAMS VRN"(w1791) -> ()
                    n3665 = local write "PrAMS Error"(w1798) -> ()
                  }
                }
              }
              event "QueryServoLevel": Value Change {
                n3666 = event-data() -> ("NewVal"=w1800:bool)  [unwired: 1 in, 4 out]
                n3667 = case shown="True" w1800 {
                  frame False {
                  }
                  frame True {
                    n3668 = local read "MessageType"() -> (w1806:cluster{string[], u32[]})
                    n3669 = control-ref of="PrAMS actif"() -> (w1805:refnum<vi>)
                    n3670 = local read "PrAMS VRN"() -> (w1803:refnum<visa-resource-name>)
                    n3671 = local read "PrAMS Error"() -> (w1804:errorcluster)
                    n3672 = local read "Signature"() -> (w1802:u32)
                    n3673 = call "SAOMM-SendGET.vi"("PRAMMS-COMM IN"=w1803, "Bool Refnum"=w1805, "MessageType"=w1806, "Signature"=w1802, "Error IN"=w1804, "Active GET"="emtGetTelescopeServoLevel" ("Active SET")) -> ("PRAMMS-COMM OUT"=w1808:refnum<visa-resource-name>, "Error OUT"=w1809:errorcluster)  [unwired: 8 in]
                    n3674 = local write "PrAMS VRN"(w1808) -> ()
                    n3675 = local write "PrAMS Error"(w1809) -> ()
                  }
                }
                n3676 = local write "QueryServoLevel"(FALSE ("QueryServoLevel")) -> ()
              }
              event "GetOptimal": Value Change {
                # "[quote=\"TELOPS\"] Ne sera pas implémenter par manque de temps ... [/quote]"
                n3677 = event-data() -> ()  [unwired: 1 in, 5 out]
                n3678 = flat-sequence {
                  tunnel: [w1813] -> w1811
                  tunnel: [w1815] -> w1810
                  tunnel: w1811 -> [w1815]
                  tunnel: w1810 -> [w1823]
                  frame #0 {
                    n3679 = local write "GetOptimal"(FALSE ("GetOptimal")) -> ()
                    n3680 = Tick Count (ms)() -> (millisecond timer value=w1813:u32)
                  }
                  frame #1 {
                    n3681 = local read "MessageType"() -> (w1817:cluster{string[], u32[]})
                    n3682 = control-ref of="PrAMS actif"() -> (w1818:refnum<vi>)
                    n3683 = local read "PrAMS Error"() -> (w1819:errorcluster)
                    n3684 = local read "PrAMS VRN"() -> (w1820:refnum<visa-resource-name>)
                    n3685 = local read "Signature"() -> (w1814:u32)
                    n3686 = call "SAOMM-SendGET.vi"("PRAMMS-COMM IN"=w1820, "Bool Refnum"=w1818, "MessageType"=w1817, "Signature"=w1814, "Error IN"=w1819, "Active GET"="emtGetOptimalExposureTime" ("Active SET")) -> ("PRAMMS-COMM OUT"=w1822:refnum<visa-resource-name>, "Error OUT"=w1821:errorcluster)  [unwired: 8 in]
                    n3687 = local write "PrAMS Error"(w1821) -> ()
                    n3688 = local write "PrAMS VRN"(w1822) -> ()
                  }
                  frame #2 {
                    "GetOptimalTime" <- w1823
                  }
                }
              }
              event "AutoCentroid": Value Change {
                # "À vérifier ...\nSemble ok : 2013-09-20"
                n3689 = event-data() -> ()  [unwired: 1 in, 5 out]
                n3690 = local write "AutoCentroid"(FALSE ("AutoCentroid")) -> ()
                n3691 = local read "XCentroid"() -> (w1845:dbl)
                n3692 = local read "YCentroid"() -> (w1846:dbl)
                n3693 = local read "XROIRef"() -> (w1829:dbl)
                n3694 = local read "YROIRef"() -> (w1828:dbl)
                n3695 = Subtract(x=w1845, y=w1829) -> (x-y=w1865:dbl)
                n3696 = Subtract(x=w1846, y=w1828) -> (x-y=w1864:dbl)
                n3697 = Round To Nearest(number=w1865) -> (nearest integer value=w1863:dbl)
                n3698 = Round To Nearest(number=w1864) -> (nearest integer value=w1862:dbl)
                n3699 = To Unsigned Word Integer(number=w1863) -> (unsigned 16bit integer=w1851:u16)
                n3700 = To Unsigned Word Integer(number=w1862) -> (unsigned 16bit integer=w1850:u16)
                n3701 = local read "Binning"() -> (w1860:u16)
                n3702 = local read "ROIWidth"() -> (w1853:u16)
                n3703 = local read "ROIHeight"() -> (w1854:u16)
                n3704 = local read "Naxis1"() -> (w1858:u16)
                n3705 = local read "Naxis2"() -> (w1857:u16)
                n3706 = local read "XROIRef"() -> (w1848:dbl)
                n3707 = local read "YROIRef"() -> (w1847:dbl)
                n3708 = Bundle("XROIRef"=w1848, "YROIRef"=w1847) -> (w1852:cluster{"XROIRef":dbl, "YROIRef":dbl})  [unwired: 1 in]
                n3709 = Bundle("Naxis1"=w1858, "Naxis2"=w1857) -> (w1859:cluster{"Naxis1":u16, "Naxis2":u16})  [unwired: 1 in]
                n3710 = Bundle("ROIWidth"=w1853, "ROIHeight"=w1854) -> (w1856:cluster{"ROIWidth":u16, "ROIHeight":u16})  [unwired: 1 in]
                n3711 = Bundle(w1851, w1850) -> (w1855:cluster{u16, u16})  [unwired: 1 in]
                n3712 = call "SAOMM-ROI_Fixer.vi"("Binning"=w1860, "Use Offset?"=TRUE, "naxis"=w1859, "ROI"=w1856, "Offset"=w1855, "Reference Pixel"=w1852) -> ("FixedOffset"=w1827:cluster{"ROIXOffset":u16, "ROIYOffset":u16}, "FixedPixel"=w1849:cluster{"PixelX":dbl, "PixelY":dbl})  [unwired: 6 in, 2 out]
                n3713 = Unbundle By Name(w1827) -> ("ROIXOffset"=w1824:u16, "ROIYOffset"=w1825:u16)
                n3714 = Unbundle By Name(w1849) -> ("PixelX"=w1837:dbl, "PixelY"=w1834:dbl)
                n3715 = local read "MessageType"() -> (w1838:cluster{string[], u32[]})
                n3716 = Bundle("ROIYOffset"=w1825, "ROIXOffset"=w1824) -> (w1826:cluster{"ROIYOffset":u16, "ROIXOffset":u16})  [unwired: 1 in]
                n3717 = control-ref of="PrAMS-ACK"() -> (w1839:refnum<vi>)
                n3718 = control-ref of="PrAMS actif"() -> (w1844:refnum<vi>)
                n3719 = local write "XReference"(w1837) -> ()
                n3720 = local write "YReference"(w1834) -> ()
                n3721 = local read "PrAMS VRN"() -> (w1843:refnum<visa-resource-name>)
                n3722 = local read "PrAMS Error"() -> (w1842:errorcluster)
                n3723 = property on="ImgArray" class="IntGraph (strict)"() -> ("Cursor.Cursor Position"=w1830:T44)  [unwired: 2 in, 2 out]
                n3724 = To Double Precision Float(number=w1824) -> (double precision float=w1835:dbl)
                n3725 = To Double Precision Float(number=w1825) -> (double precision float=w1836:dbl)
                n3726 = Add(x=w1836, y=w1837) -> (x+y=w1833:dbl)
                n3727 = Add(x=w1835, y=w1834) -> (x+y=w1832:dbl)
                n3728 = call "SAOMM-UpdateROI.vi"("PRAMMS-COMM IN"=w1843, "Active Refnum"=w1844, "PrAMS-ACK"=w1839, "MessageType"=w1838, "Error IN"=w1842, "Position"=w1826) -> ("PRAMMS-COMM OUT"=w1841:refnum<visa-resource-name>, "Error OUT"=w1840:errorcluster)  [unwired: 7 in, 1 out]
                n3729 = Bundle(cluster=w1830, "Cursor X"=w1833, "Cursor Y"=w1832) -> (w1831:T44)
                n3730 = local write "PrAMS Error"(w1840) -> ()
                n3731 = local write "PrAMS VRN"(w1841) -> ()
